vi "setMinValue.vi"(8 "error in (no error)":errorcluster, 10 "minValue":dbl, 11 "ACNET Devices in":refnum<class "ACNET Device.lvclass">) -> (0 "error out":errorcluster, 3 "ACNET Devices out":refnum<class "ACNET Device.lvclass">)   [LabVIEW 2013, in "ACNET Monitor.lvlib" / "ACNET Device.lvclass"]
uses:
  ACNET Device.lvclass
  ACNET Device.lvclass/ACNET Device.ctl
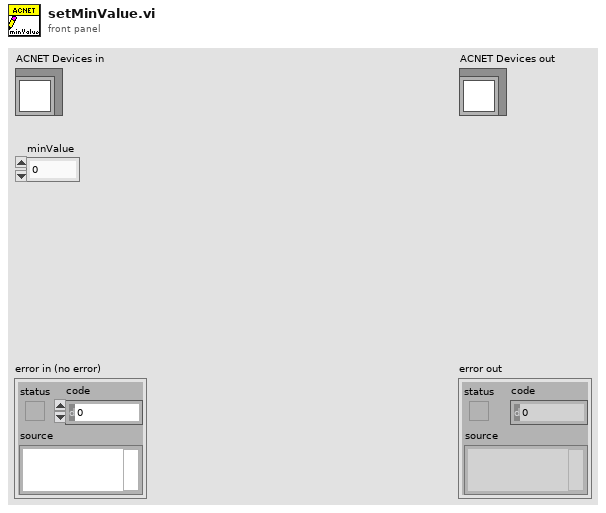
[diagram p1: front panel]
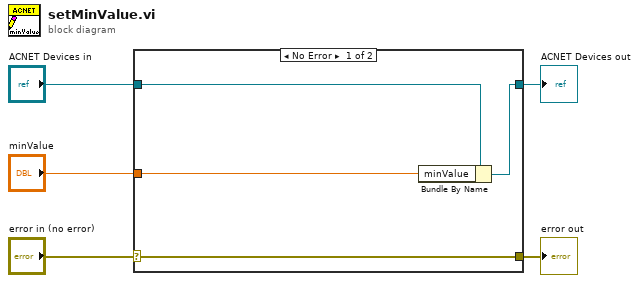
[diagram p0: block diagram]
diagram:
  n1 = case shown="No Error" "error in (no error)" {
    selector: "error in (no error)" -> [w9 w10]
    tunnel: [w9 w10] -> w4
    tunnel: [w7 w11] -> w2
    tunnel: "ACNET Devices in" -> [w8 w11]
    tunnel: "minValue" -> [w6 _]
    frame No Error {
      n2 = Bundle By Name(cluster=w8, "minValue"=w6) -> (w7:refnum<class "ACNET Device.lvclass">)
    }
    frame Error {
    }
  }
  "error out" <- w4
  "ACNET Devices out" <- w2
